vi "Test Pass if in Set.vi"(8 "error in (no error)":errorcluster, 11 "Dummy In":refnum<class "Example Test Case.lvclass">) -> (0 "error out":errorcluster, 3 "Dummy Out":refnum<class "Example Test Case.lvclass">)   [LabVIEW 2020, in "Example Test Case.lvclass"]
doc: "Failing test"
uses:
  Example Test Case.lvclass
  C:/git/astemes-lunit/source/API/LUnit Test Case/LUnit Test Case.lvclass
  Core/LUnit Test Case/LUnit Test Case.lvclass/LUnit Test Case.ctl
  f7599997-06c6-4163-a399-60519fa8dddf.vi
  Core/LUnit Test Case/Assertions/Pass If.vi
  Core/LUnit Test Case/Private/Append Fail Result.vi
  Core/LUnit Test Case/Private/Append Pass Result.vi
  Core/LUnit Test Case/Private/Run In UI.vi
  <vilib>/Utility/error.llb/Clear Errors.vi
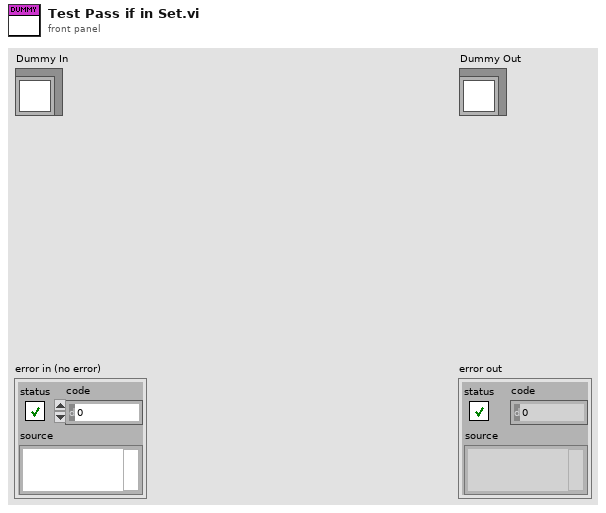
[diagram p1: front panel]
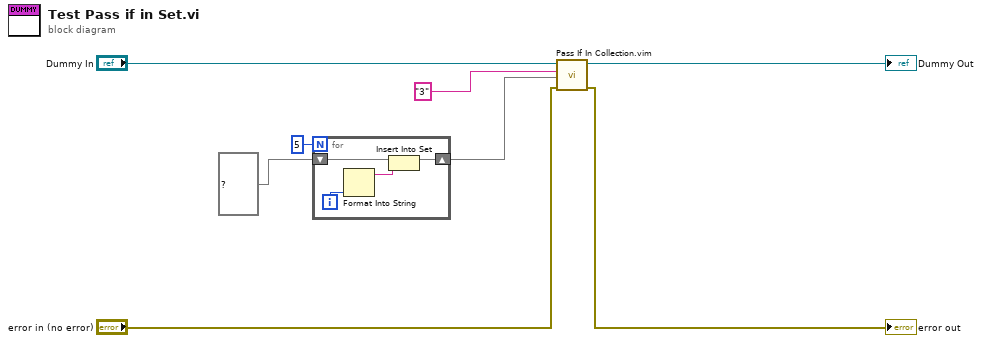
[diagram p0: block diagram]
diagram:
  n1 = for {
    N: 5 -> [_]
    shift-right: [w9] -> w1
    shift-left: set{string} {} ("map") -> [w12]
    i -> [w11]
    n2 = Format Into String(w11) -> (resulting string=w10:string)  [unwired: 3 in, 1 out]
    n3 = Insert Into Set(10:w10, 11:w12) -> (3:w9:set{string})  [unwired: 1 out]
  }
  n4 = call "Pass If In Collection.vim"("error in (no error)"="error in (no error)", "Collection"=w1, "Expected Element"="3", "LUnit Test Case In"="Dummy In") -> ("error out"=→"error out":errorcluster, "LUnit Test Case Out"=→"Dummy Out":refnum<class "Example Test Case.lvclass">)  [unwired: 6 in]
